vi "test_check_gpx-file.vi"() -> ()   [LabVIEW 2019]
uses:
  Patrolrobot/Subvi/Gmap/dll/GMap.NET.WindowsForms.dll
  Ctrl/cmd_common.ctl
  Gmap/gmap_fgv-cmd.ctl
  Gmap/marker_info.ctl
panel:
  in  "waypoint conversion":bool
  out "XY 그래프":cluster{"X":dbl, "Y":dbl}[](graph)
  in  "path":path=path "C:/AGV/Config/waypoint/gpx/1course-2.gpx"
  in  "GPX file load":bool
  in  "Lat":dbl=37.369722329400446 format="%.11f"
  in  "Lon Dbclk":dbl format="%.11f"
  in  "Lat Dbclk":dbl format="%.11f"
  in  "Lon":dbl=126.72567486763 format="%.11f"
  in  "GMapControl":refnum<k24>(container)
  in  "PinDropMrkr":T1(ring)=enum."red_dot" caption="Pin Drop Marker"
  in  "zoom":dbl(slide)=18.0 scale=3.0..20.0
  in  "stop":bool=TRUE
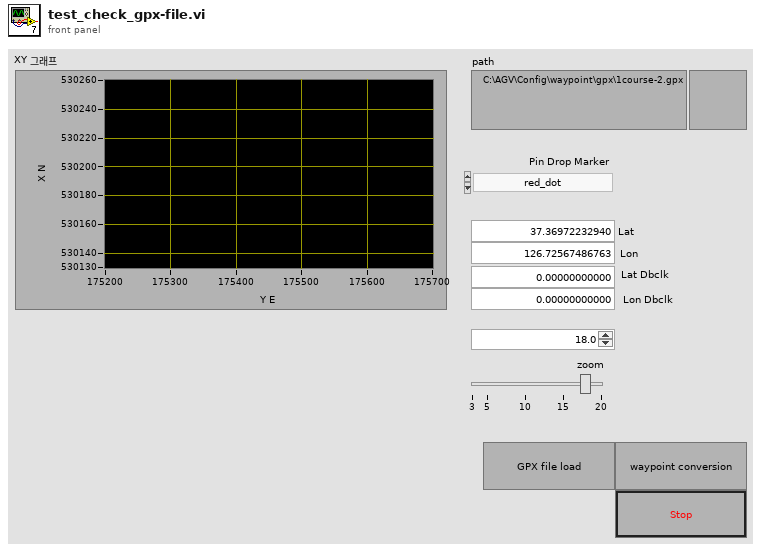
[diagram p1: front panel]
types:
  T1 = enum16{"none", "arrow", "blue", "blue_small", "blue_dot", "blue_pushpin", "brown_small", "gray_small", "green", "green_small", "green_dot", "green_pushpin", "green_big_go", "yellow", "yellow_small", "yellow_dot", "yellow_big_pause", "yellow_pushpin", "lightblue", "lightblue_dot", "lightblue_pushpin", "orange", "orange_small", "orange_dot", "pink", "pink_dot", "pink_pushpin", "purple", "purple_small", "purple_dot", "purple_pushpin", "red", "red_small", "red_dot", "red_pushpin", "red_big_stop", "black_small", "white_small"}
  T2 = typedef "cmd_common.ctl" = enum16{"read", "write"}
  T3 = cluster{"Lat":refnum<vi>, "Lon":refnum<vi>, "Lat Dbclk":refnum<vi>, "Lon Dbclk":refnum<vi>, "zoom":refnum<vi>, "PinDropMrkr":refnum<vi>}
  T4 = typedef "gmap_fgv-cmd.ctl" = enum16{"marker type change", "save_image", "coll of points", "zoom n center markers", "add overlay reference", "read", "zoom", "set position by keyword", "set map provider", "map provider update", "create", "add marker", "clear marker", "close"}
  T5 = typedef "marker_info.ctl" = cluster{"arrLatLngActv":dbl[], "type":i32}
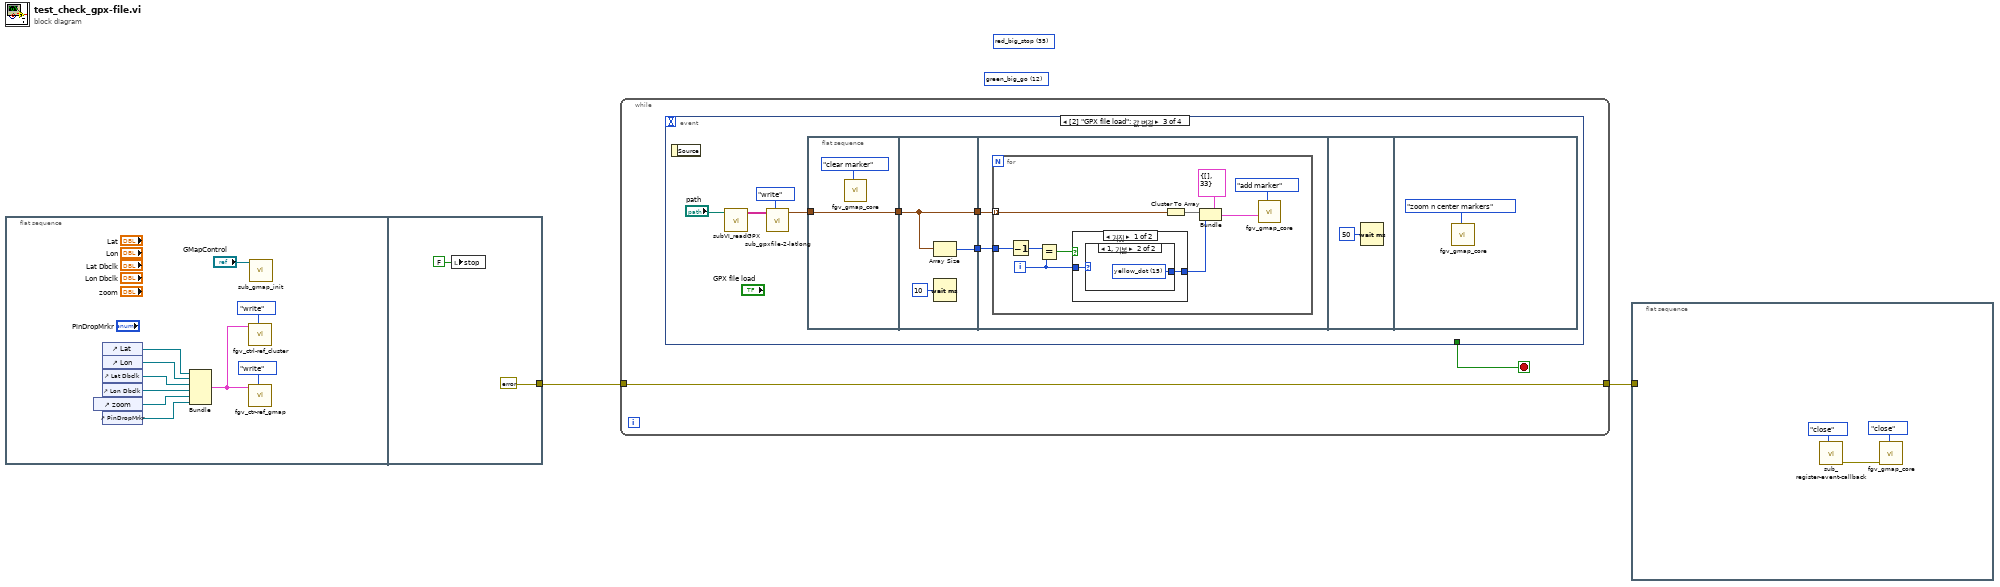
[diagram p0: block diagram]
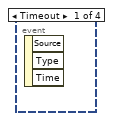
[diagram p2: hidden frame]
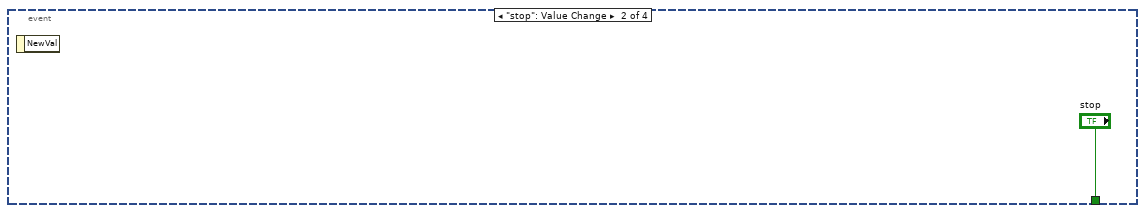
[diagram p3: hidden frame]
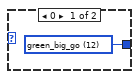
[diagram p4: hidden frame]
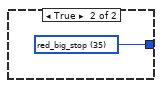
[diagram p5: hidden frame]
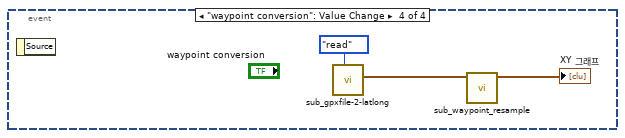
[diagram p6: hidden frame]
diagram:
  (unwired) 12 items=["none", "arrow", "blue", "blue_small", "blue_dot", "blue_pushpin", "brown_small", "gray_small", "green", "green_small", "green_dot", "green_pushpin", "green_big_go", "yellow", "yellow_small", "yellow_dot", "yellow_big_pause", "yellow_pushpin", "lightblue", "lightblue_dot", "lightblue_pushpin", "orange", "orange_small", "orange_dot", "pink", "pink_dot", "pink_pushpin", "purple", "purple_small", "purple_dot", "purple_pushpin", "red", "red_small", "red_dot", "red_pushpin", "red_big_stop", "black_small", "white_small"] ("type")
  (unwired) 35 items=["none", "arrow", "blue", "blue_small", "blue_dot", "blue_pushpin", "brown_small", "gray_small", "green", "green_small", "green_dot", "green_pushpin", "green_big_go", "yellow", "yellow_small", "yellow_dot", "yellow_big_pause", "yellow_pushpin", "lightblue", "lightblue_dot", "lightblue_pushpin", "orange", "orange_small", "orange_dot", "pink", "pink_dot", "pink_pushpin", "purple", "purple_small", "purple_dot", "purple_pushpin", "red", "red_small", "red_dot", "red_pushpin", "red_big_stop", "black_small", "white_small"] ("type")
  n1 = flat-sequence {
    tunnel: [errorcluster {"status"=FALSE, "code"=0, "source"=""} ("error out")] -> w2
    frame #0 {
      n2 = control-ref of="zoom"() -> (w6:refnum<vi>)
      n3 = control-ref of="Lat"() -> (w10:refnum<vi>)
      n4 = control-ref of="Lon"() -> (w9:refnum<vi>)
      n5 = control-ref of="Lat Dbclk"() -> (w8:refnum<vi>)
      n6 = control-ref of="Lon Dbclk"() -> (w7:refnum<vi>)
      n7 = control-ref of="PinDropMrkr"() -> (w5:refnum<vi>)
      n8 = Bundle("Lat"=w10, "Lon"=w9, "Lat Dbclk"=w8, "Lon Dbclk"=w7, "zoom"=w6, "PinDropMrkr"=w5) -> (w3:T3)  [unwired: 1 in]
      n9 = call "fgv_ctrl-ref_cluster.vi"("cmd"=enum16{"read", "write"}."write", "ref"=w3) -> ()  [unwired: 9 in, 1 out]
      n10 = call "fgv_ctr-ref_gmap.vi"("cmd"=cmd_common."write", "ref in"=w3) -> ()  [unwired: 9 in, 1 out]
      n11 = call "sub_gmap_init.vi"("GMapControl"="GMapControl") -> ()  [unwired: 10 in, 1 out]
    }
    frame #1 {
      n12 = local write "stop"(FALSE ("정지")) -> ()
    }
  }
  n13 = while {
    tunnel: w2 -> [w16]
    tunnel: [w16] -> w1
    stop <- w15 stop-if-true
    n14 = event shown="[2] \"GPX file load\": 값 변경" {
      selector: _ -> [_ _ _ _]
      dyn-events: _ -> [_ _ _ _]
      timeout: _ -> [_ _ _ _]
      tunnel: [_ "stop" _ _] -> w15
      event Timeout {
        n15 = event-data() -> ()  [unwired: 1 in, 3 out]
      }
      event "stop": Value Change {
        n16 = event-data() -> ()  [unwired: 1 in, 1 out]
      }
      event "GPX file load": Value Change {
        n17 = event-data() -> ()  [unwired: 1 in, 1 out]
        n18 = call "subVI_readGPX.vi"("file (use dialog)"="path") -> ("wpt Array"=w23:string[][])  [unwired: 8 in]
        n19 = call "sub_gpxfile-2-latlong.vi"("cmd"=cmd_common."write", "wpt Array"=w23) -> ("latlong"=w20:cluster{dbl, dbl}[])  [unwired: 8 in, 1 out]
        n20 = flat-sequence {
          tunnel: [w25] -> w21
          tunnel: w20 -> [w25]
          tunnel: [w28] -> w22
          tunnel: w21 -> [w28]
          tunnel: [w27] -> w19
          tunnel: w22 -> [w31]
          tunnel: w19 -> [w30]
          frame #0 {
            n21 = call "fgv_gmap_core.vi"("cmd"=gmap_fgv-cmd."clear marker") -> ()  [unwired: 7 in, 4 out]
          }
          frame #1 {
            n22 = Array Size(array=w28) -> (size(s)=w27:i32)
            n23 = Wait (ms)(milliseconds to wait=u32 10 ("대기 시간 (ms)")) -> ()  [unwired: 1 out]
          }
          frame #2 {
            n24 = for {
              tunnel: w31 -> [w37] mode=indexing
              tunnel: w30 -> [w35]
              i -> [w34]
              n25 = Decrement(x=w35) -> (x-1=w33:i32)
              n26 = Equal?(x=w33, y=w34) -> (x = y?=w32:bool)
              n27 = case shown="거짓" w32 {
                tunnel: [w43 w46] -> w36
                tunnel: w34 -> [w42 _]
                frame False {
                  n28 = case shown="1, 기본" w42 {
                    tunnel: [w44 w45] -> w43
                    frame 0 {
                      w44 = 12 items=["none", "arrow", "blue", "blue_small", "blue_dot", "blue_pushpin", "brown_small", "gray_small", "green", "green_small", "green_dot", "green_pushpin", "green_big_go", "yellow", "yellow_small", "yellow_dot", "yellow_big_pause", "yellow_pushpin", "lightblue", "lightblue_dot", "lightblue_pushpin", "orange", "orange_small", "orange_dot", "pink", "pink_dot", "pink_pushpin", "purple", "purple_small", "purple_dot", "purple_pushpin", "red", "red_small", "red_dot", "red_pushpin", "red_big_stop", "black_small", "white_small"] ("type")
                    }
                    frame 1, Default {
                      w45 = 15 items=["none", "arrow", "blue", "blue_small", "blue_dot", "blue_pushpin", "brown_small", "gray_small", "green", "green_small", "green_dot", "green_pushpin", "green_big_go", "yellow", "yellow_small", "yellow_dot", "yellow_big_pause", "yellow_pushpin", "lightblue", "lightblue_dot", "lightblue_pushpin", "orange", "orange_small", "orange_dot", "pink", "pink_dot", "pink_pushpin", "purple", "purple_small", "purple_dot", "purple_pushpin", "red", "red_small", "red_dot", "red_pushpin", "red_big_stop", "black_small", "white_small"] ("type")
                    }
                  }
                }
                frame True {
                  w46 = 35 items=["none", "arrow", "blue", "blue_small", "blue_dot", "blue_pushpin", "brown_small", "gray_small", "green", "green_small", "green_dot", "green_pushpin", "green_big_go", "yellow", "yellow_small", "yellow_dot", "yellow_big_pause", "yellow_pushpin", "lightblue", "lightblue_dot", "lightblue_pushpin", "orange", "orange_small", "orange_dot", "pink", "pink_dot", "pink_pushpin", "purple", "purple_small", "purple_dot", "purple_pushpin", "red", "red_small", "red_dot", "red_pushpin", "red_big_stop", "black_small", "white_small"] ("type")
                }
              }
              n29 = Cluster To Array(cluster=w37) -> (array=w40:dbl[])
              n30 = Bundle(cluster=T5 {"arrLatLngActv"=[], "type"=33} ("marker_info"), "arrLatLngActv"=w40, "type"=w36) -> (w38:T5)
              n31 = call "fgv_gmap_core.vi"("cmd"=gmap_fgv-cmd."add marker", "marker_info"=w38) -> ()  [unwired: 6 in, 4 out]
            }
          }
          frame #3 {
            n32 = Wait (ms)(milliseconds to wait=u32 50 ("대기 시간 (ms)")) -> ()  [unwired: 1 out]
          }
          frame #4 {
            n33 = call "fgv_gmap_core.vi"("cmd"=gmap_fgv-cmd."zoom n center markers") -> ()  [unwired: 7 in, 4 out]
          }
        }
      }
      event "waypoint conversion": Value Change {
        n34 = event-data() -> ()  [unwired: 1 in, 1 out]
        n35 = call "sub_gpxfile-2-latlong.vi"("cmd"=cmd_common."read") -> ("tm"=w49:cluster{"Y(E)":dbl, "X(N)":dbl}[])  [unwired: 9 in, 1 out]
        n36 = call "sub_waypoint_resample.vi"("line point"=w49) -> ("interpolate 1d array"=→"XY 그래프":cluster{dbl, dbl}[])  [unwired: 9 in, 1 out]
      }
    }
  }
  n37 = flat-sequence {
    tunnel: w1 -> [_]
    frame #0 {
      n38 = call "sub_register-event-callback.vi"("cmd"=enum16{"register", "close"}."close") -> ("error out"=w52:errorcluster)  [unwired: 10 in]
      n39 = call "fgv_gmap_core.vi"("cmd"=gmap_fgv-cmd."close", "error in"=w52) -> ()  [unwired: 6 in, 4 out]
    }
  }
